vi "Read Stamp Tool Vacuum.vi"(8 "error in":errorcluster, 11 "Gantry in":refnum<class "Gantry Class.lvclass">) -> (0 "error out":errorcluster, 2 "On/Off":bool, 3 "Gantry out":refnum<class "Gantry Class.lvclass">)   [LabVIEW 2011, in "Gantry Class.lvclass"]
uses:
  Gantry Class.lvclass
  WorkTable Class/WorkTable Class.lvclass
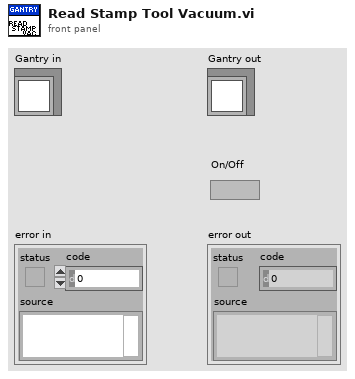
[diagram p1: front panel]
types:
  T1 = typedef "Worktable_Stamps.ctl" = cluster{"Stamp Slots":cluster{"Stamp State":enum16{"Empty", "Populated", "Used"}, "Stamp Type":enum16{"Stamp 1", "Stamp 2", "Stamp 3", "Stamp 4"}, "Location/Orientation":T2}[], "Vacuum Channel":u8}
  T2 = typedef "Position_Orientation.ctl" = cluster{"Center":refnum<class "Vec3d Class.lvclass">, "Orientation":refnum<class "Orient3d Class.lvclass">}
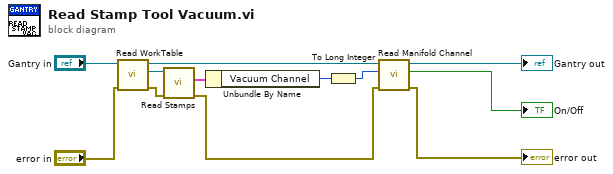
[diagram p0: block diagram]
diagram:
  n1 = call-dynamic "Read WorkTable.vi"("error in"="error in", "Gantry Class in"="Gantry in") -> ("error out"=w5:errorcluster, "WorkTable Class.lvclass"=w7:refnum<class "WorkTable Class.lvclass">, "Gantry Class out"=w8:refnum<class "Gantry Class.lvclass">)  [unwired: 7 in]
  n2 = call-dynamic "Read Stamps.vi"("error in (no error)"=w5, "WorkTable Class in"=w7) -> ("error out"=w4:errorcluster, "Stamps"=w6:T1)  [unwired: 7 in, 1 out]
  n3 = Unbundle By Name(w6) -> ("Vacuum Channel"=w3:u8)
  n4 = To Long Integer(number=w3) -> (32bit integer=w2:i32)
  n5 = call-dynamic "Read Manifold Channel.vi"("error in"=w4, "Manifold Channel"=w2, "Gantry in"=w8) -> ("error out"=→"error out":errorcluster, "On/Off"=→"On/Off":bool, "Gantry out"=→"Gantry out":refnum<class "Gantry Class.lvclass">)  [unwired: 6 in]
